vi "滤波.vi"(1 "X":dbl[](array[numeric]) caption="输入信号数组") -> (0 "Filtered X":dbl[](array[numeric]) caption="滤波信号数组")   [LabVIEW 2018]
uses:
  <vilib>/Analysis/3filter.llb/Equi-Ripple BandStop (DBL).vi
  <vilib>/Analysis/NI_AALBase.lvlib
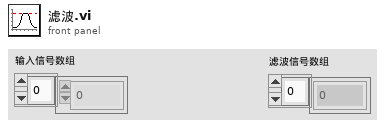
[diagram p1: front panel]
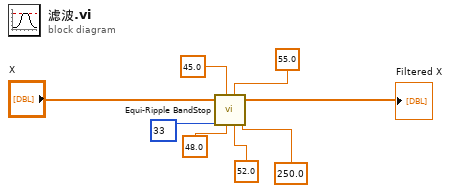
[diagram p0: block diagram]
diagram:
  n1 = call-poly <vilib>:"Equi-Ripple BandStop.vi"("X"="X", "lower pass freq"=45.0, "# of taps"=33, "lower stop freq"=48.0, "higher pass freq"=55.0, "higher stop freq"=52.0, "sampling freq: fs"=250.0) -> ("Filtered X"=→"Filtered X":dbl[])  [unwired: 1 in, 1 out]
